vi "Card Test.vi"() -> ()   [LabVIEW 2019]
doc: "This example program initialize the card and perform the hardware card \ntest with a configurable test level (0-3), and it also utilizes sensors on the\nhardware to measure the desired sensor value.\n\nNote: Card Test Level 3 takes a few minutes to complete and must not be\nrun when connected to an active databus as it will transmit onto the bus."
uses:
  <instrlib>/BTICardLib/Public/Controls/Card Test Level.ctl
  <instrlib>/BTICardLib/Public/Controls/Sensor Type.ctl
  <instrlib>/BTICardLib/Private/Initialize By Card Number and Core Number.vi
  <instrlib>/BTICardLib/BTICardLV.lvlib
panel:
  out "Sensor Type":T1=1 items=["SENSOR_NONE", "SENSOR_TEMP", "SENSOR_VOLTAGE", "SENSOR_CURRENT"]
  in  "Sensor":T2(ring)=enum."FPGA"
  out "Measured Sensor Value":string="42.0 C"
  out "Card Test Result":string="PASS"
  in  "Test Level":T3=3 items=["TEST_LEVEL0", "TEST_LEVEL1", "TEST_LEVEL2", "TEST_LEVEL3"]
  out "Error":errorcluster
  in  "Card Number":i32
  in  "Core Number":i32
  # "Card Test"
  # "©2016 Astronics Ballard Technology"
  # "This example program initialize the card and perform the hardware card \ntest with a configurable test level (0-3), and it also utilizes sensors on the\nhardware to measure the desired sensor value.\n\nNote: Card Test Level 3 takes a few minutes to complete and must not be\nrun when connected to an active databus as it will transmit onto the bus."
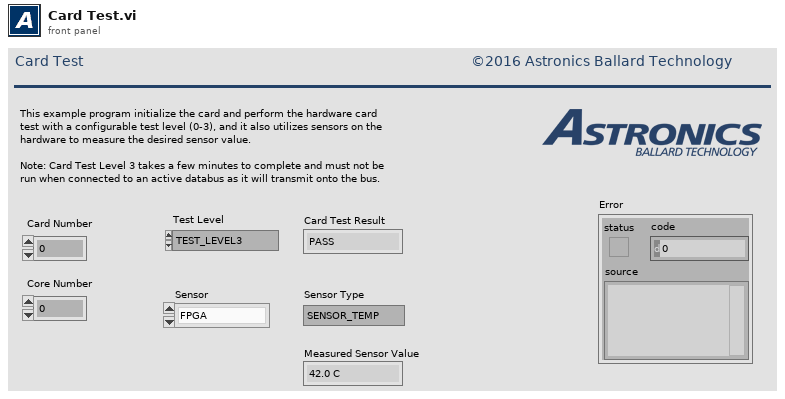
[diagram p1: front panel]
types:
  T1 = typedef "BTICardLV.lvlib/Sensor Type.ctl" = u32
  T2 = enum16{"PCB", "FPGA", "I/O Module", "Power Supply"}
  T3 = typedef "BTICardLV.lvlib/Card Test Level.ctl" = u32
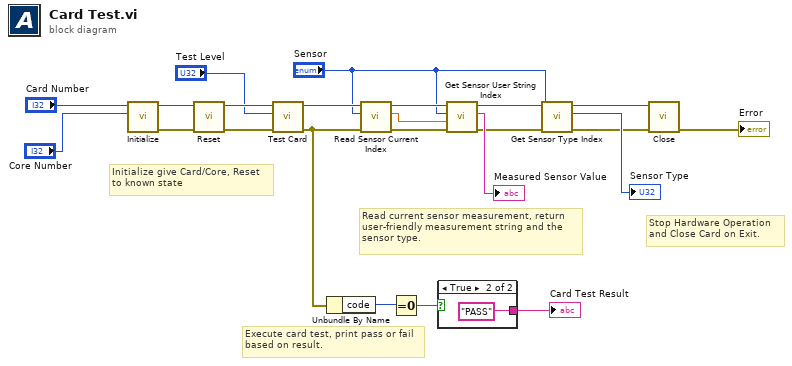
[diagram p0: block diagram]
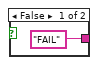
[diagram p2: hidden frame]
diagram:
  # "Initialize give Card/Core, Reset\nto known state"
  # "Execute card test, print pass or fail\nbased on result."
  # "Read current sensor measurement, return\nuser-friendly measurement string and the\nsensor type."
  # "Stop Hardware Operation\nand Close Card on Exit."
  n1 = call-poly <instrlib>:"Initialize.vi"("core number"="Core Number", "card number"="Card Number") -> ("error out"=w19:errorcluster, "core handle out"=w20:u64)  [unwired: 8 in]
  n2 = call <instrlib>:"Reset.vi"("error in (no error)"=w19, "core handle in"=w20) -> ("error out"=w17:errorcluster, "core handle out"=w18:u64)  [unwired: 8 in]
  n3 = call <instrlib>:"Test Card.vi"("error in (no error)"=w17, "test level"="Test Level", "core handle in"=w18) -> ("error out"=w11:errorcluster, "core handle out"=w5:u64)  [unwired: 7 in]
  n4 = Unbundle By Name(w11) -> ("code"=w12:i32)
  n5 = call <instrlib>:"Read Sensor Current Index.vi"("error in (no error)"=w11, "index"="Sensor", "core handle in"=w5) -> ("error out"=w10:errorcluster, "now"=w8:dbl, "core handle out"=w9:u64)  [unwired: 6 in]
  n6 = Equal To 0?(x=w12) -> (x = 0?=w13:bool)
  n7 = case shown="True" w13 {
    tunnel: ["FAIL" "PASS"] -> w14
    frame False {
    }
    frame True {
    }
  }
  "Card Test Result" <- w14
  n8 = call <instrlib>:"Get Sensor User String Index.vi"("error in (no error)"=w10, "value"=w8, "index"="Sensor", "core handle in"=w9) -> ("error out"=w4:errorcluster, "user string"=→"Measured Sensor Value":string, "core handle out"=w6:u64)  [unwired: 5 in]
  n9 = call <instrlib>:"Get Sensor Type Index.vi"("error in (no error)"=w4, "index"="Sensor", "core handle in"=w5) -> ("error out"=w1:errorcluster, "sensor type"=→"Sensor Type":T1)  [unwired: 6 in, 1 out]
  n10 = call <instrlib>:"Close.vi"("error in (no error)"=w1, "core handle in"=w6) -> ("error out"=→"Error":errorcluster)  [unwired: 8 in, 1 out]
